vi "Store Value in TDMS.vi"(5 "Replace name with prefix (FALSE = append)":bool, 6 "Value":variant, 7 "Prefix":string, 8 "Error In":errorcluster, 9 "channel name":string, 10 "group name":string, 11 "tdms file":refnum<k34>) -> (0 "Error Out":errorcluster, 1 "channel name out":string, 2 "group name out":string, 3 "tdms file out":refnum<k34>)   [LabVIEW 2024]
uses:
  <vilib>/Utility/Data Type/Type Definitions/Data Type.ctl
  <vilib>/Utility/Data Type/NI_Data Type.lvlib
  <userlib>/_OpenG.lib/lvdata/lvdata.llb/openg_variant.lvlib
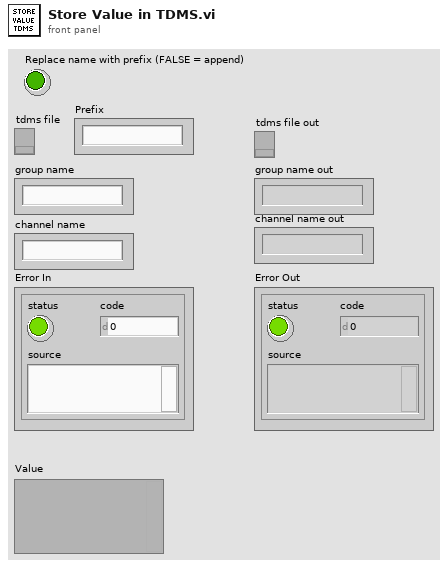
[diagram p1: front panel]
types:
  T1 = typedef "NI_Data Type.lvlib/Data Type.ctl" = enum8{"Invalid Type", "Void", "I8", "I16", "I32", "I64", "U8", "U16", "U32", "U64", "Single Float", "Double Float", "Extended Float", "Single Complex", "Double Complex", "Extended Complex", "Enum U8", "Enum U16", "Enum U32", "Enum U64", "Single Float With Unit", "Double Float With Unit", "Extended Float With Unit", "Single Complex with Unit", "Double Complex with Unit", "Extended Complex with Unit", "Boolean", "String", "Path", "Picture", "Tag", "Array", "Cluster", "Variant", "LV Variant", "Waveform", "Timestamp", "Digital Waveform", "Digital Data", "ExpressData", "Refnum", "External Data", "VI", "Poly VI", "LabVIEW Class Instance", "Fixed Point", "Set Collection", "Map Collection"}
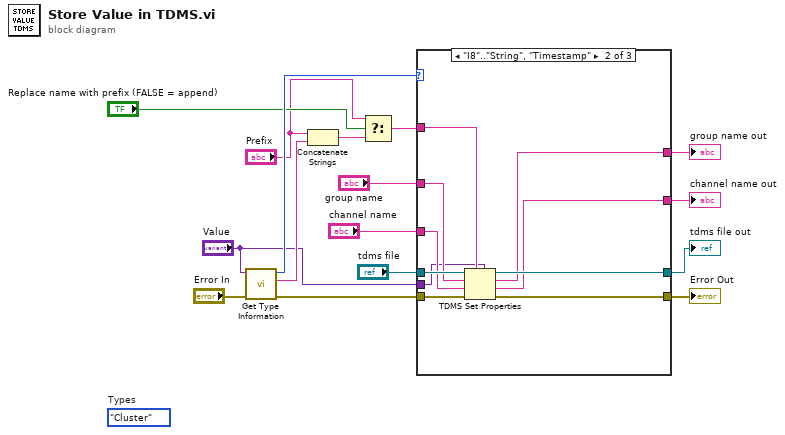
[diagram p0: block diagram]
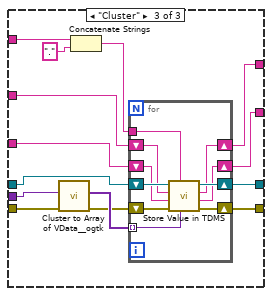
[diagram p3: hidden frame]
diagram:
  (unwired) Data_Type."Cluster"  # Types
  n1 = call <vilib>:"Get Type Information.vi"("error in (no error)"="Error In", "variant"="Value") -> ("error out"=w7:errorcluster, "name"=w9:string, "type"=w6:T1)  [unwired: 5 in, 2 out]
  n2 = Concatenate Strings("Prefix", w9) -> (w2:string)
  n3 = Select(t="Prefix", s="Replace name with prefix (FALSE = append)", f=w2) -> (s? t:f=w1:string)
  n4 = case shown="\"I8\"..\"String\", \"Timestamp\"" w6 {
    tunnel: "tdms file" -> [w20 w30 w44]
    tunnel: [w20 w29 w38] -> w15
    tunnel: "group name" -> [w18 w28 w43]
    tunnel: "channel name" -> [w17 w27 w42]
    tunnel: [w17 w26 w40] -> w12
    tunnel: [w18 w25 w41] -> w11
    tunnel: w7 -> [w19 w24 w32]
    tunnel: [w19 w23 w39] -> w10
    tunnel: w1 -> [_ w22 w37]
    tunnel: "Value" -> [_ w21 w34]
    frame "Invalid Type", Default {
    }
    frame "I8".."String", "Timestamp" {
      n5 = TDMS Set Properties(5:w21, 7:w22, 8:w24, 9:w27, 10:w28, 11:w30) -> (0:w23:errorcluster, 1:w26:string, 2:w25:string, 3:w29:refnum<k34>)
    }
    frame "Cluster" {
      n6 = call <userlib>:"Cluster to Array of VData__ogtk.vi"("error in (no error)"=w32, "Cluster"=w34) -> ("error out"=w31:errorcluster, "Array of VData"=w33:variant[])  [unwired: 8 in]
      n7 = Concatenate Strings(w37, "." ("string")) -> (w35:string)
      n8 = for {
        shift-right: [w51] -> w39
        shift-left: w31 -> [w53]
        shift-right: [w52] -> w38
        shift-left: w44 -> [w54]
        shift-right: [w47] -> w41
        shift-left: w43 -> [w50]
        shift-right: [w48] -> w40
        shift-left: w42 -> [w49]
        tunnel: w33 -> [w46] mode=indexing
        tunnel: w35 -> [w45]
        n9 = call "Store Value in TDMS.vi"("Value"=w46, "Prefix"=w45, "Error In"=w53, "channel name"=w49, "group name"=w50, "tdms file"=w54) -> ("Error Out"=w51:errorcluster, "channel name out"=w48:string, "group name out"=w47:string, "tdms file out"=w52:refnum<k34>)  [unwired: 2 in]
      }
    }
  }
  "Error Out" <- w10
  "tdms file out" <- w15
  "channel name out" <- w12
  "group name out" <- w11
